vi "initialize_data_log.vi"(7 "Overwrite?":bool, 8 "error in (no error)":errorcluster, 9 "Initialization Data":variant, 10 "Path":path, 11 "hdf5_photon_record_log in":refnum<class "hdf5_photon_record_log.lvclass">) -> (0 "error out":errorcluster, 3 "hdf5_photon_record_log out":refnum<class "hdf5_photon_record_log.lvclass">)   [LabVIEW 2015, in "hdf5_photon_record_log.lvclass"]
uses:
  hdf5_photon_record_log.lvclass
  hydraharp_panel/hpanel_acq_modes.ctl
  hdf5_photon_record_log.lvclass/hdf5_photon_record_log.ctl
  <vilib>/UPVI/lvhdf5/file.llb/LVH5F Operation.ctl
  <vilib>/UPVI/lvhdf5/dataset.llb/LVH5D Operation.ctl
  <vilib>/UPVI/lvhdf5/property.llb/LVH5PClassId.ctl
  <vilib>/UPVI/lvhdf5/library.llb/HDF5 Ref.ctl
  <vilib>/UPVI/lvhdf5/datatype.llb/LVH5Tcreate_dataset_type (Variant).vi
  <vilib>/UPVI/lvhdf5/datatype.llb/LVH5Tcreate_dataset_type.xnode
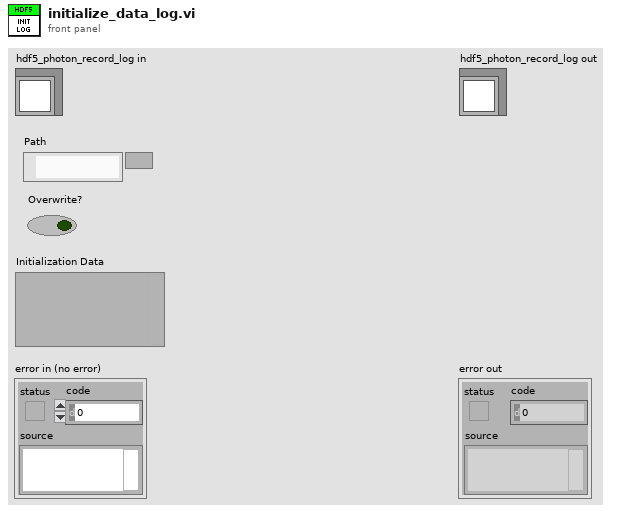
[diagram p1: front panel]
types:
  T1 = typedef "hpanel_acq_modes.ctl" = u16
  T2 = typedef "LVH5D Operation.ctl" = enum16{"open", "replace", "create", "open or create", "create or replace", "create or replace with confirmation"}
  T3 = typedef "LVH5PClassId.ctl" = enum32{"H5P_ROOT", "H5P_OBJECT_CREATE", "H5P_FILE_CREATE", "H5P_FILE_ACCESS", "H5P_DATASET_CREATE", "H5P_DATASET_ACCESS", "H5P_DATASET_XFER", "H5P_FILE_MOUNT", "H5P_GROUP_CREATE", "H5P_GROUP_ACCESS", "H5P_DATATYPE_CREATE", "H5P_DATATYPE_ACCESS", "H5P_STRING_CREATE", "H5P_ATTRIBUTE_CREATE", "H5P_OBJECT_COPY", "H5P_LINK_CREATE", "H5P_LINK_ACCESS"}
  T4 = typedef "LVH5F Operation.ctl" = enum16{"open", "open or create", "create or replace", "create or replace (with confirmation)", "create", "open (read only)"}
  T5 = typedef "HDF5 Ref.ctl" = refnum<k1>
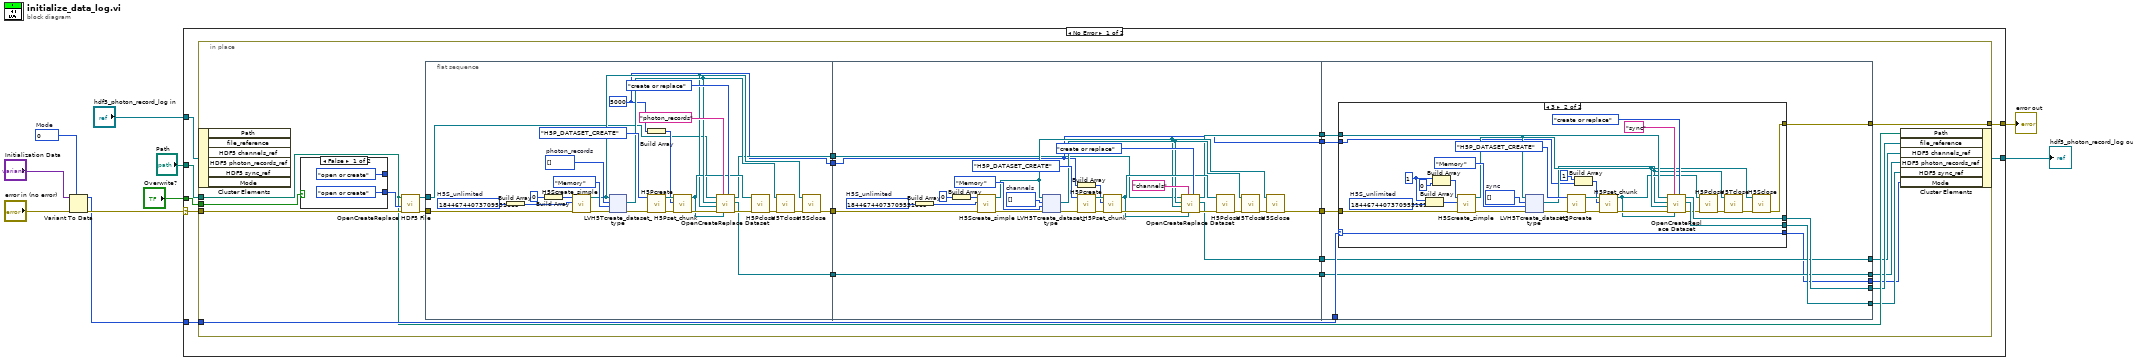
[diagram p0: block diagram]
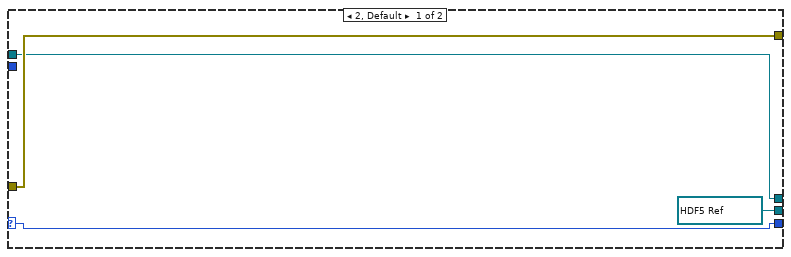
[diagram p2: hidden frame]
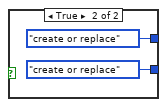
[diagram p3: hidden frame]
diagram:
  w3 = T1 0 items=["T2"=2, "T3"=3]  # Mode
  n1 = Variant To Data(error in="error in (no error)", type=w3, Variant="Initialization Data") -> (data=w2:T1, error out=w4:errorcluster)
  n2 = case shown="No Error" w4 {
    selector: w4 -> [w13 w215]
    tunnel: "Path" -> [w17 _]
    tunnel: "Overwrite?" -> [w16 _]
    tunnel: [w15 w216] -> w8
    tunnel: "hdf5_photon_record_log in" -> [w14 w216]
    tunnel: w2 -> [w12 _]
    tunnel: [w11 w215] -> w1
    frame No Error {
      n3 = in-place {
        in-place-border: w17 -> [w23]
        in-place-border: w16 -> [w39]
        in-place-border: w13 -> [w37]
        in-place-border: w12 -> [w25]
        in-place-border: [w24] -> w11
        n4 = in-place-cluster #1(w14) -> ()  [unwired: 6 out]
        n5 = case shown="False" w39 {
          tunnel: [LVH5F_Operation."open or create" ("function (open or create)") LVH5F_Operation."create or replace" ("function (open or create)")] -> w38
          tunnel: [LVH5D_Operation."open or create" ("operation (open or create)") LVH5D_Operation."create or replace" ("operation (open or create)")] -> _
          frame False {
          }
          frame True {
          }
        }
        n6 = call <vilib>:"OpenCreateReplace HDF5 File.vi"("error in (no error)"=w37, "function (open or create)"=w38, "path"=w23) -> ("error out"=w36:errorcluster, "HDF5 Ref out"=w35:T5)  [unwired: 5 in]
        n7 = flat-sequence {
          tunnel: w36 -> [w45]
          tunnel: w35 -> [w44]
          tunnel: [w43] -> w34
          tunnel: [w42] -> w33
          tunnel: [w41] -> w32
          tunnel: [w40] -> w31
          tunnel: w34 -> [w95]
          tunnel: w33 -> [w96]
          tunnel: w32 -> [w93]
          tunnel: w31 -> [w97]
          tunnel: [w95] -> w30
          tunnel: [w94] -> w29
          tunnel: [w93] -> w28
          tunnel: [w92] -> w27
          tunnel: [w91] -> w26
          tunnel: w30 -> [w145]
          tunnel: w29 -> [w152]
          tunnel: w28 -> [w151]
          tunnel: w27 -> [w144]
          tunnel: w26 -> [w150]
          tunnel: w25 -> [w149]
          tunnel: [w148] -> w24
          tunnel: [w147] -> w22
          tunnel: [w146] -> w19
          tunnel: [w145] -> w20
          tunnel: [w144] -> w21
          tunnel: [w143] -> w18
          frame #0 {
            w41 = 5000
            w57 = u64[] []  # photon_records
            w61 = u64 18446744073709551615  # H5S_unlimited
            n8 = Build Array(w61) -> (w60:u64[])
            n9 = Build Array(u64 0 ("element")) -> (w58:u64[])
            n10 = call <vilib>:"H5Screate_simple.vi"("error in (no error)"=w45, "Maximum Dimensions (unlimited)"=w60, "Dimensions"=w58) -> ("error out"=w66:errorcluster, "HDF5 Ref out"=w46:T5)  [unwired: 5 in]
            n11 = xnode "LVH5Tcreate_dataset_type"("HDF5 Location Ref"=w46, "Type"=enum16{"File", "Memory"}."Memory", "error in (no error)"=w66, "Data"=w57) -> ("HDF5 Type Ref"=w48:T5, "error out"=w63:errorcluster)  [unwired: 2 in, 3 out]
            n12 = Build Array(w41) -> (w54:i32[])
            n13 = call <vilib>:"H5Pcreate.vi"("error in (no error)"=w63, "Property List Class"=LVH5PClassId."H5P_DATASET_CREATE") -> ("error out"=w64:errorcluster, "HDF5 Property List Ref"=w65:T5)  [unwired: 6 in]
            n14 = call <vilib>:"H5Pset_chunk.vi"("error in (no error)"=w64, "Dimensions"=w54, "HDF5 Property Ref"=w65) -> ("error out"=w62:errorcluster, "HDF5 Ref out"=w47:T5)  [unwired: 5 in]
            n15 = call <vilib>:"OpenCreateReplace Dataset.vi"("operation (open or create)"=LVH5D_Operation."create or replace", "HDF5 Property List Ref"=w47, "Dataset Path"="photon_records" ("string"), "error in (no error)"=w62, "HDF5 Dataspace Ref"=w46, "HDF5 Datatype Ref"=w48, "HDF5 Ref"=w44) -> ("error out"=w49:errorcluster, "HDF5 Dataset Ref"=w43:T5, "HDF5 Ref out"=w42:T5)  [unwired: 2 in]
            n16 = call <vilib>:"H5Pclose.vi"("error in (no error)"=w49, "HDF5 Property Ref"=w47) -> ("error out"=w51:errorcluster)  [unwired: 7 in]
            n17 = call <vilib>:"H5Tclose.vi"("error in (no error)"=w51, "HDF5 Datatype Ref"=w48) -> ("error out"=w50:errorcluster)  [unwired: 7 in]
            n18 = call <vilib>:"H5Sclose.vi"("error in (no error)"=w50, "HDF5 Dataspace Ref"=w46) -> ("error out"=w40:errorcluster)  [unwired: 7 in]
          }
          frame #1 {
            w101 = u64 18446744073709551615  # H5S_unlimited
            w113 = u8[] []  # channels
            n19 = Build Array(w101) -> (w99:u64[])
            n20 = Build Array(u64 0 ("element")) -> (w98:u64[])
            n21 = call <vilib>:"H5Screate_simple.vi"("error in (no error)"=w97, "Maximum Dimensions (unlimited)"=w99, "Dimensions"=w98) -> ("error out"=w118:errorcluster, "HDF5 Ref out"=w102:T5)  [unwired: 5 in]
            n22 = xnode "LVH5Tcreate_dataset_type"("HDF5 Location Ref"=w102, "Type"=enum16{"File", "Memory"}."Memory", "error in (no error)"=w118, "Data"=w113) -> ("HDF5 Type Ref"=w103:T5, "error out"=w115:errorcluster)  [unwired: 2 in, 3 out]
            n23 = Build Array(w93) -> (w110:i32[])
            n24 = call <vilib>:"H5Pcreate.vi"("error in (no error)"=w115, "Property List Class"=LVH5PClassId."H5P_DATASET_CREATE") -> ("error out"=w116:errorcluster, "HDF5 Property List Ref"=w117:T5)  [unwired: 6 in]
            n25 = call <vilib>:"H5Pset_chunk.vi"("error in (no error)"=w116, "Dimensions"=w110, "HDF5 Property Ref"=w117) -> ("error out"=w114:errorcluster, "HDF5 Ref out"=w104:T5)  [unwired: 5 in]
            n26 = call <vilib>:"OpenCreateReplace Dataset.vi"("operation (open or create)"=LVH5D_Operation."create or replace", "HDF5 Property List Ref"=w104, "Dataset Path"="channels" ("string"), "error in (no error)"=w114, "HDF5 Dataspace Ref"=w102, "HDF5 Datatype Ref"=w103, "HDF5 Ref"=w96) -> ("error out"=w105:errorcluster, "HDF5 Dataset Ref"=w92:T5, "HDF5 Ref out"=w94:T5)  [unwired: 2 in]
            n27 = call <vilib>:"H5Pclose.vi"("error in (no error)"=w105, "HDF5 Property Ref"=w104) -> ("error out"=w107:errorcluster)  [unwired: 7 in]
            n28 = call <vilib>:"H5Tclose.vi"("error in (no error)"=w107, "HDF5 Datatype Ref"=w103) -> ("error out"=w106:errorcluster)  [unwired: 7 in]
            n29 = call <vilib>:"H5Sclose.vi"("error in (no error)"=w106, "HDF5 Dataspace Ref"=w102) -> ("error out"=w91:errorcluster)  [unwired: 7 in]
          }
          frame #2 {
            n30 = case shown="3" w149 {
              selector: w149 -> [w153 w166]
              tunnel: w150 -> [w156 w170]
              tunnel: [w156 w161] -> w148
              tunnel: w152 -> [w155 w169]
              tunnel: [w155 w168] -> w147
              tunnel: [w154 w167] -> w146
              tunnel: [w153 w166] -> w143
              tunnel: w151 -> [_ w157]
              frame 2, Default {
                w154 = T5 refnum items=["HDF5 Ref"] ("HDF5 Dataset Ref")
              }
              frame 3 {
                w176 = u64[] []  # sync
                w179 = u64 1 ("element")
                w181 = u64 18446744073709551615  # H5S_unlimited
                n31 = Build Array(w179, w181) -> (w180:u64[])
                n32 = Build Array(w179, u64 0 ("element")) -> (w177:u64[])
                n33 = call <vilib>:"H5Screate_simple.vi"("error in (no error)"=w170, "Maximum Dimensions (unlimited)"=w180, "Dimensions"=w177) -> ("error out"=w186:errorcluster, "HDF5 Ref out"=w160:T5)  [unwired: 5 in]
                n34 = xnode "LVH5Tcreate_dataset_type"("HDF5 Location Ref"=w160, "Type"=enum16{"File", "Memory"}."Memory", "error in (no error)"=w186, "Data"=w176) -> ("HDF5 Type Ref"=w158:T5, "error out"=w183:errorcluster)  [unwired: 2 in, 3 out]
                n35 = call <vilib>:"H5Pcreate.vi"("error in (no error)"=w183, "Property List Class"=LVH5PClassId."H5P_DATASET_CREATE") -> ("error out"=w184:errorcluster, "HDF5 Property List Ref"=w185:T5)  [unwired: 6 in]
                n36 = Build Array(1 ("element"), w157) -> (w172:i32[])
                n37 = call <vilib>:"H5Pset_chunk.vi"("error in (no error)"=w184, "Dimensions"=w172, "HDF5 Property Ref"=w185) -> ("error out"=w182:errorcluster, "HDF5 Ref out"=w159:T5)  [unwired: 5 in]
                n38 = call <vilib>:"OpenCreateReplace Dataset.vi"("operation (open or create)"=LVH5D_Operation."create or replace", "HDF5 Property List Ref"=w159, "Dataset Path"="sync" ("string"), "error in (no error)"=w182, "HDF5 Dataspace Ref"=w160, "HDF5 Datatype Ref"=w158, "HDF5 Ref"=w169) -> ("error out"=w162:errorcluster, "HDF5 Dataset Ref"=w167:T5, "HDF5 Ref out"=w168:T5)  [unwired: 2 in]
                n39 = call <vilib>:"H5Pclose.vi"("error in (no error)"=w162, "HDF5 Property Ref"=w159) -> ("error out"=w164:errorcluster)  [unwired: 7 in]
                n40 = call <vilib>:"H5Tclose.vi"("error in (no error)"=w164, "HDF5 Datatype Ref"=w158) -> ("error out"=w163:errorcluster)  [unwired: 7 in]
                n41 = call <vilib>:"H5Sclose.vi"("error in (no error)"=w163, "HDF5 Dataspace Ref"=w160) -> ("error out"=w161:errorcluster)  [unwired: 7 in]
              }
            }
          }
        }
        n42 = in-place-cluster #1("Path"=w23, "file_reference"=w22, "HDF5 channels_ref"=w21, "HDF5 photon_records_ref"=w20, "HDF5 sync_ref"=w19, "Mode"=w18) -> (w15:refnum<class "hdf5_photon_record_log.lvclass">)
      }
    }
    frame Error {
    }
  }
  "error out" <- w1
  "hdf5_photon_record_log out" <- w8
